vi "Create Laplacian 64f.vi"(8 "Error In":errorcluster, 9 "Dimension":T1={"Depth"=1, "Height"=1, "Width"=1} {"Width" min=1; "Height" min=1; "Depth" min=1}, 10 "Memory Object":T2 {"Dimension"."Width" min=1; "Dimension"."Height" min=1; "Dimension"."Depth" min=1}, 11 "Device In":T3) -> (0 "Error Out":errorcluster, 1 "Dimension Out":T1={"Depth"=1, "Height"=1, "Width"=1} {"Width" min=1; "Height" min=1; "Depth" min=1}, 3 "Laplacian Out":T6 {"Laplacian Out"."Dimension"."Width" min=1; "Laplacian Out"."Dimension"."Height" min=1; "Laplacian Out"."Dimension"."Depth" min=1})   [LabVIEW 2012, in "OpenCLV x64.lvlib"]
doc: "Creates a Laplacian Object and allocates space for the destination memory object. Either the dimension or a prior memory object must be provided."
uses:
  OpenCLV x64.lvlib
  Controls/Device ID.ctl
  User Controls/Array Dimensions.ctl
  Controls/Laplacian Object.ctl
  Controls/Program Handle.ctl
  Controls/Memory Object.ctl
  Controls/Memory ID.ctl
  Controls/Memory Type.ctl
  Allocate Memory/AllocateMemory_64f.vi
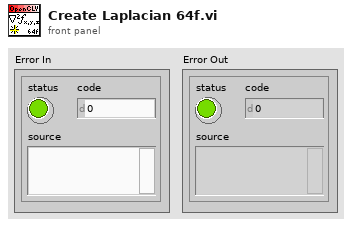
[diagram p1: front panel]
types:
  T1 = typedef "Array Dimensions.ctl" = cluster{"Depth":u64, "Height":u64, "Width":u64}
  T2 = typedef "OpenCLV x64.lvlib/Memory Object.ctl" = cluster{"Device ID":T3, "Memeroy ID":T4, "Dimension":T1, "Memory Type":T5}
  T3 = typedef "OpenCLV x64.lvlib/Device ID.ctl" = u64
  T4 = typedef "OpenCLV x64.lvlib/Memory ID.ctl" = u64
  T5 = typedef "OpenCLV x64.lvlib/Memory Type.ctl" = enum16{"32f", "u8", "i8", "u16", "i16", "u32", "i32", "64f"}
  T6 = typedef "OpenCLV x64.lvlib/Laplacian Object.ctl" = cluster{"Device Out":T3, "Program Handle":T7, "Laplacian Out":T2}
  T7 = typedef "OpenCLV x64.lvlib/Program Handle.ctl" = u64
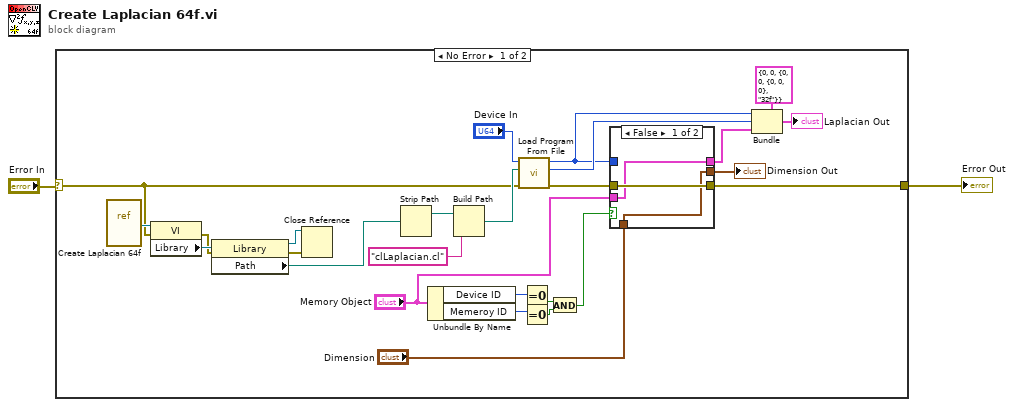
[diagram p0: block diagram]
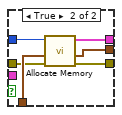
[diagram p2: hidden frame]
diagram:
  n1 = case shown="No Error" "Error In" {
    selector: "Error In" -> [w4 w38]
    tunnel: [w7 w38] -> w1
    frame No Error {
      n2 = vi-ref "Create Laplacian 64f.vi"() -> (w24:refnum<vi>)
      n3 = property class="VI"(reference=w24, error in=w4) -> (error out=w3:errorcluster, "Library"=w23:refnum<vi>)  [unwired: 1 out]
      n4 = property class="Library"(reference=w23, error in=w3) -> (reference out=w8:refnum<vi>, error out=w9:errorcluster, "Path"=w22:path)
      n5 = Close Reference(reference=w8, error in (no error)=w9) -> ()  [unwired: 1 out]
      n6 = Strip Path(path=w22) -> (stripped path=w28:path)  [unwired: 1 out]
      n7 = Unbundle By Name("Memory Object") -> ("Device ID"=w17:T3, "Memeroy ID"=w16:T4)
      n8 = Build Path(base path=w28, name or relative path="clLaplacian.cl") -> (appended path=w26:path)
      n9 = call "Load Program From File.vi"("Error In"=w4, "Program Path"=w26, "Device In"="Device In") -> ("Error Out"=w15:errorcluster, "Program Handle"=w19:T7, "Device Out"=w14:T3)  [unwired: 6 in]
      n10 = Equal To 0?(x=w17) -> (x = 0?=w12:bool)
      n11 = Equal To 0?(x=w16) -> (x = 0?=w18:bool)
      n12 = And(x=w12, y=w18) -> (x .and. y?=w10:bool)
      n13 = case shown="False" w10 {
        tunnel: "Dimension" -> [w29 w37]
        tunnel: w15 -> [w31 w36]
        tunnel: [w30 w35] -> w13
        tunnel: [w31 w34] -> w7
        tunnel: w14 -> [_ w33]
        tunnel: "Memory Object" -> [w30 _]
        tunnel: [w29 w32] -> w5
        frame False {
        }
        frame True {
          n14 = call-poly "Allocate Memory.vi"("Error In"=w36, "Dimension"=w37, "Device In"=w33) -> ("Error Out"=w34:errorcluster, "Dimensions Out"=w32:T1, "Memory Object"=w35:T2)  [unwired: 6 in]
        }
      }
      "Dimension Out" <- w5
      n15 = Bundle(cluster=T6 {"Device Out"=0, "Program Handle"=0, "Laplacian Out"={"Device ID"=0, "Memeroy ID"=0, "Dimension"={"Depth"=0, "Height"=0, "Width"=0}, "Memory Type"=enum."32f"}} ("Laplacian Object"), "Device Out"=w14, "Program Handle"=w19, "Laplacian Out"=w13) -> (→"Laplacian Out":T6)
    }
    frame Error {
    }
  }
  "Error Out" <- w1
